vi "Dispense glue sequence.vi"(6 "Syringe map":dbl[](array[numeric]), 8 "error in (no error)":errorcluster, 10 "Assembly Tray map":dbl[][](array[numeric]), 11 "Assembly Run in":refnum<class "Assembly Run.lvclass">) -> (0 "error out":errorcluster, 3 "Assembly Run out":refnum<class "Assembly Run.lvclass">)   [LabVIEW 2020, in "Assembly Run.lvclass"]
uses:
  Assembly Run.lvclass
  Workspace/Fixture Enum.ctl
  Workspace/Fixture.lvclass
  Routine/Routine Enum.ctl
  Routine/Routine.lvclass
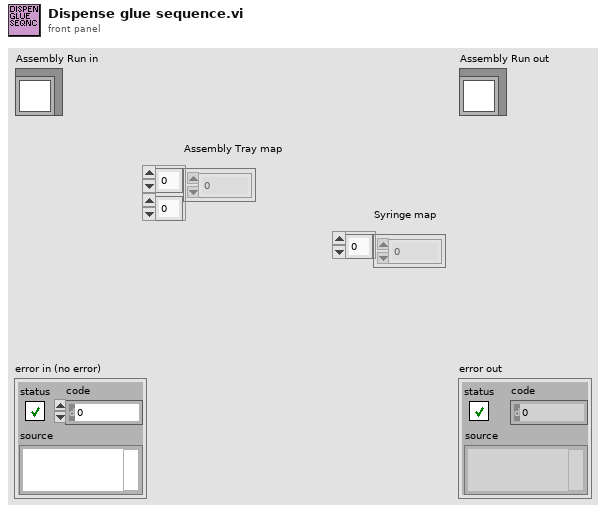
[diagram p1: front panel]
types:
  T1 = typedef "Routine.lvclass/Routine Enum.ctl" = enum16{"Primary Pick Up", "Pick Up All", "Put Down Secondary", "Put Down All", "Release Syringe", "Secondary Pick Up", "Secure Syringe", "Dispense on Plate", "Dispense on Kapton", "Dispense on Sensor"}
  T2 = typedef "Fixture.lvclass/Fixture Enum.ctl" = enum16{"Assembly Tray", "Syringe Space", "Component", "Pick Up Tool", "Current Position"}
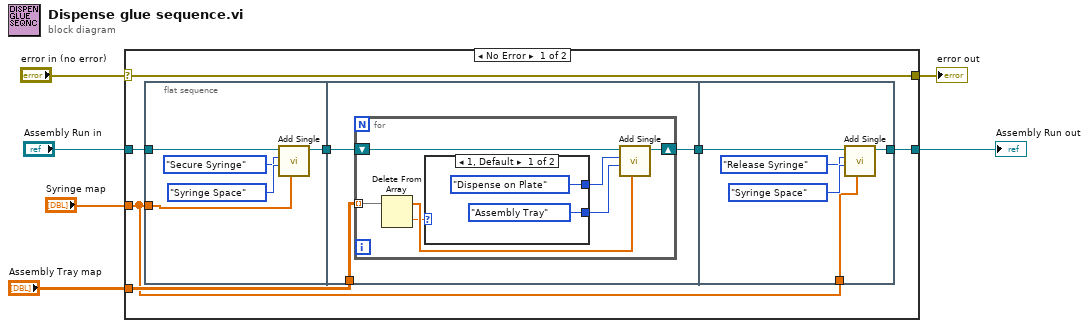
[diagram p0: block diagram]
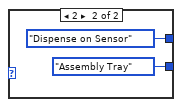
[diagram p2: hidden frame]
diagram:
  n1 = case shown="No Error" "error in (no error)" {
    selector: "error in (no error)" -> [w13 w39]
    tunnel: [w13 w39] -> w5
    tunnel: [w9 w38] -> w3
    tunnel: "Assembly Run in" -> [w10 w38]
    tunnel: "Assembly Tray map" -> [w8 _]
    tunnel: "Syringe map" -> [w7 _]
    frame No Error {
      n2 = flat-sequence {
        tunnel: [w16] -> w12
        tunnel: w10 -> [w15]
        tunnel: w7 -> [w14]
        tunnel: w12 -> [w20]
        tunnel: [w21] -> w11
        tunnel: w8 -> [w19]
        tunnel: w11 -> [w35]
        tunnel: [w34] -> w9
        tunnel: w7 -> [w33]
        frame #0 {
          n3 = call-dynamic "Add Single.vi"("Gantry map"=w14, "Fixture"=Fixture_Enum."Syringe Space", "Routine"=Routine_Enum."Secure Syringe" ("Routine 2"), "UI in"=w15) -> ("UI out"=w16:refnum<class "Assembly Run.lvclass">)  [unwired: 5 in, 1 out]
        }
        frame #1 {
          n4 = for {
            shift-right: [w26] -> w21
            shift-left: w20 -> [w25]
            tunnel: w19 -> [w24] mode=indexing
            n5 = Delete From Array(array=w24) -> (deleted portion=w22:dbl, array with subset deleted=w23:dbl[])  [unwired: 2 in]
            n6 = case shown="1, Default" w22 {
              tunnel: [Fixture_Enum."Assembly Tray" ("Fixture") Fixture_Enum."Assembly Tray" ("Fixture")] -> w27
              tunnel: [Routine_Enum."Dispense on Plate" ("Routine 2") Routine_Enum."Dispense on Sensor" ("Routine 2")] -> w28
              frame 1, Default {
              }
              frame 2 {
              }
            }
            n7 = call-dynamic "Add Single.vi"("Gantry map"=w23, "Fixture"=w27, "Routine"=w28, "UI in"=w25) -> ("UI out"=w26:refnum<class "Assembly Run.lvclass">)  [unwired: 5 in, 1 out]
          }
        }
        frame #2 {
          n8 = call-dynamic "Add Single.vi"("Gantry map"=w33, "Fixture"=Fixture_Enum."Syringe Space", "Routine"=Routine_Enum."Release Syringe" ("Routine 2"), "UI in"=w35) -> ("UI out"=w34:refnum<class "Assembly Run.lvclass">)  [unwired: 5 in, 1 out]
        }
      }
    }
    frame Error {
    }
  }
  "error out" <- w5
  "Assembly Run out" <- w3
